vi "Get Data Type of TDMS Property.vi"() -> ()   [LabVIEW 2023]
doc: "This example demonstrates how to get the data type of a property on TDMS objects (channel/group/root) using TDMS Get Property Data Type VI.\n\nRefer to the block diagram of this VI for information about using the TDMS Get Property Data Type VI."
panel:
  out "Data Type of Property":u16 format="%02x"
  # "Overview: Demonstrates how to retrieve the data type of a property on TDMS objects with the TDMS Get Property Data Type VI. \nInstructions:\n1. Run the VI.  \n2. Delete the .tdms file (located at [LabVIEW Data]\\Example Property Data Type.tdms) when you are done."
  # "Note: The mapping between Data Type and numeric type code is defined in LabVIEW Help. Select Help > LabVIEW Help and navigate to Contents > Fundamentals > How LabVIEW Stores Data in Memory > Concepts > Type Descriptors for more information."
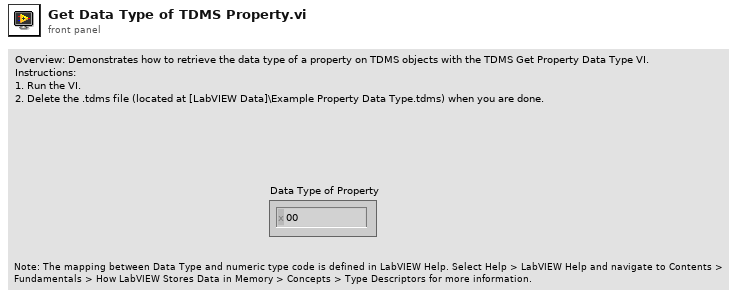
[diagram p1: front panel]
types:
  T1 = enum16{"open", "open or create", "create or replace", "create", "open (read-only)"}
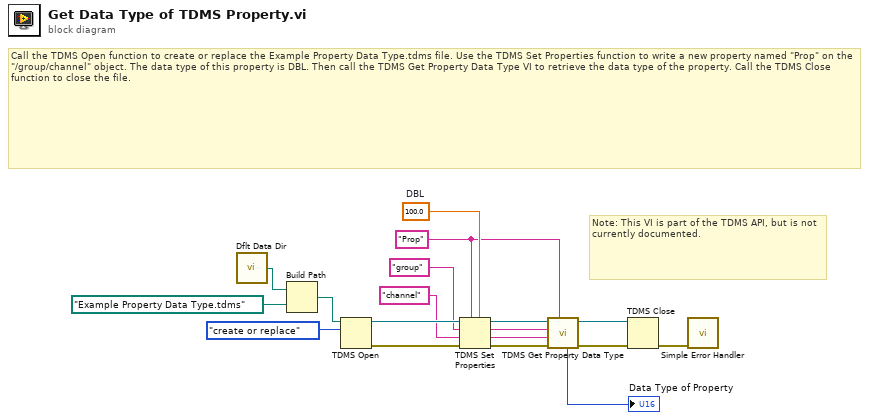
[diagram p0: block diagram]
diagram:
  w12 = 100.0  # DBL
  w5 = "Prop"
  # "Note: This VI is part of the TDMS API, but is not currently documented."
  # "Call the TDMS Open function to create or replace the Example Property Data Type.tdms file. Use the TDMS Set Properties function to write a new property named \"Prop\" on the \"/group/channel\" object. The data type of this property is DBL. Then call the TDMS Get Property Data Type VI to retrieve the data type of the property. Call the TDMS Close function to close the file."
  n1 = call <vilib>:"Dflt Data Dir.vi"() -> ("App:Default Data Directory"=w2:path)
  n2 = Build Path(base path=w2, name or relative path=path "Example Property Data Type.tdms" ("Application Directory")) -> (appended path=w18:path)
  n3 = TDMS Open(10:T1."create or replace" ("operation (0:open)"), 11:w18) -> (0:w15:errorcluster, 3:w16:refnum<k34>)  [unwired: 5 in]
  n4 = TDMS Set Properties(5:w12, 7:w5, 8:w15, 9:"channel" ("group name"), 10:"group" ("group name"), 11:w16) -> (0:w11:errorcluster, 1:w6:string, 2:w7:string, 3:w9:refnum<k34>)
  n5 = call <vilib>:"TDMS Get Property Data Type.vi"("property name"=w5, "error in (no error)"=w11, "channel name"=w6, "group name"=w7, "tdms file"=w9) -> ("error out"=w10:errorcluster, "tdms file out"=w8:refnum<k34>, "data type"=→"Data Type of Property":u16)  [unwired: 2 in, 2 out]
  n6 = TDMS Close(8:w10, 11:w8) -> (0:w4:errorcluster)  [unwired: 1 out]
  n7 = call <vilib>:"Simple Error Handler.vi"("error in (no error)"=w4) -> ()  [unwired: 4 in, 5 out]
